vi "Write Table Control.vi"(8 "error in (no error)":errorcluster, 10 "Table Control":refnum<vi>, 11 "Geocoding in":refnum<class "Geocoding.lvclass">) -> (0 "error out":errorcluster, 3 "Geocoding out":refnum<class "Geocoding.lvclass">)   [LabVIEW 2025, in "Geocoding Actor.lvlib" / "Geocoding.lvclass"]
uses:
  Geocoding.lvclass
  Geocoding.lvclass/Geocoding.ctl
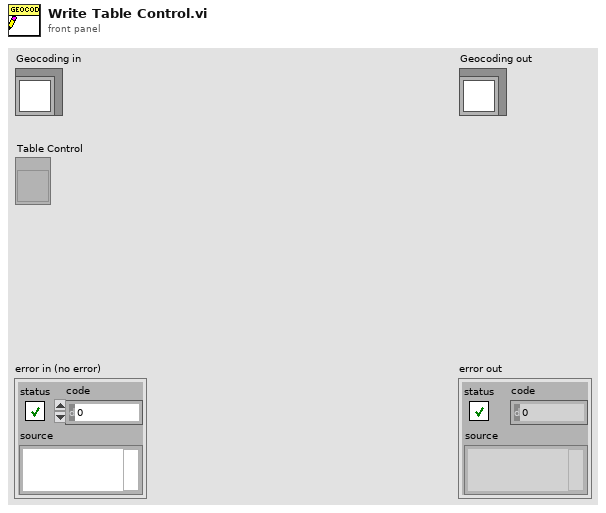
[diagram p1: front panel]
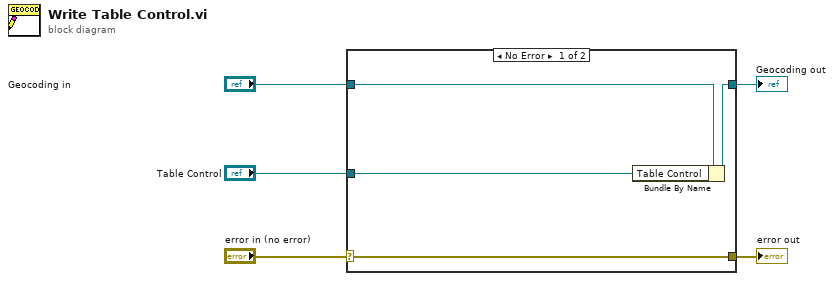
[diagram p0: block diagram]
diagram:
  n1 = case shown="No Error" "error in (no error)" {
    selector: "error in (no error)" -> [w9 w10]
    tunnel: [w9 w10] -> w4
    tunnel: [w7 w11] -> w2
    tunnel: "Geocoding in" -> [w8 w11]
    tunnel: "Table Control" -> [w6 _]
    frame No Error {
      n2 = Bundle By Name(cluster=w8, "Table Control"=w6) -> (w7:refnum<class "Geocoding.lvclass">)
    }
    frame Error {
    }
  }
  "error out" <- w4
  "Geocoding out" <- w2
